vi "Chasis_Omni_Ultimate.vi"() -> ()   [LabVIEW 2010, in "Fiel Orientation Compass.lvrbt"]
uses:
  Fiel Orientation Compass.lvrbt
  <vilib>/NXT/HiTechnic/HiTechnic Controls/HiTechnic Port.ctl
  <vilib>/NXT/Block Support/NXT_InputPort.ctl
  <vilib>/NXT/NXTIO Xnodes/AddressXNode/NXTIOAddress.xnode
  <vilib>/NXT/Subs/MotorXNode.DC Motor Type.ctl
  Desktop/Teleop1.lvrbt_2012_01_27_1934/Teleop1/Teleop1.lvrbt
  <vilib>/NXT/Subs/MotorXNode.1DCMotor.ctl
  <vilib>/NXT/Subs/LVHSConnector.ctl
  <vilib>/NXT/NXTIO Xnodes/NXTIOXNode/NXTIO.xnode
  <vilib>/FTC/FTC Interpret Motor Power From Right X Axis.vi
  <vilib>/FTC/FTC Interpret Motor Power From Left Y Axis.vi
  <vilib>/FTC/FTC Interpret Motor Power From Left X Axis.vi
  <vilib>/NXT/Dual Mode Library/prims/inRangeAndCoerce/inRangeAndCoerce_float.vi
  <vilib>/NXT/NXTIO Xnodes/NXTIONodeSubVIs/TETRIX IO Move DC Motors.vi
panel:
  out "LEFT Y":i8
  out "LEFT X":i8
  out "y'":dbl
  out "x'":dbl
  out "INITIAL":dbl
  # "This VI was generated based on your configuration in the Remote Control Editor. You may modify the code as needed for your robot. To test this program for an FTC match, return to the Remote Control Editor, select the \"Run Program\" tab, and choose \"FTC Game\"."
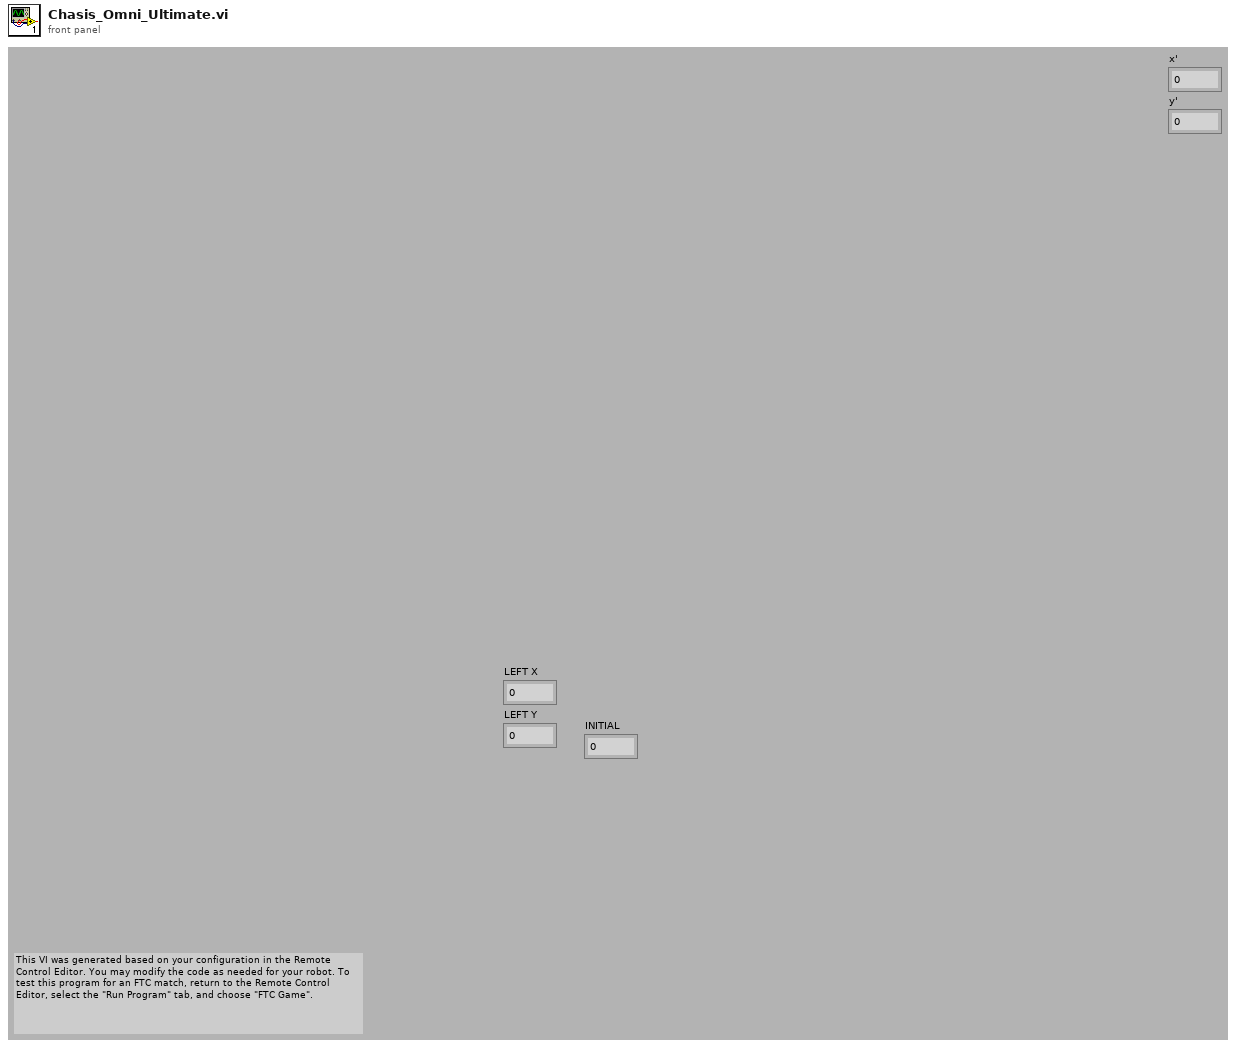
[diagram p1: front panel]
types:
  T1 = typedef "HiTechnic Port.ctl" = cluster{"Port":T2, "MUX Port":u8}
  T2 = typedef "NXT_InputPort.ctl" = u8
  T3 = typedef "LVHSConnector.ctl" = cluster{"Hardware":string, "Flattened String":string}
  T4 = typedef "FTC ControllerState.ctl" = cluster{"Left X":i8, "Left Y":i8, "Right X":i8, "Right Y":i8, "Button Encoding 9-12":u8, "Button Encoding 1-8":u8, "POV":T5}
  T5 = typedef "FTC POVState.ctl" = i8
  T6 = typedef "FTC ButtonEventType.ctl" = enum16{"Pressed", "Released"}
  T7 = cluster{"Button ID":enum16{"None", "Button 1", "Button 2", "Button 3", "Button 4", "Button 5", "Button 6", "Button 7", "Button 8", "Button 9", "Button 10", "Button 11", "Button 12", "POV Up", "POV Up Right", "POV Right", "POV Down Right", "POV Down", "POV Down Left", "POV Left", "POV Up Left"}, "Event Type":T6}[]
  T8 = enum16{"None", "Button 1", "Button 2", "Button 3", "Button 4", "Button 5", "Button 6", "Button 7", "Button 8", "Button 9", "Button 10", "Button 11", "Button 12", "POV Up", "POV Up Right", "POV Right", "POV Down Right", "POV Down", "POV Down Left", "POV Left", "POV Up Left"}
  T9 = typedef "MotorXNode.DC Motor Type.ctl" = enum16{"DC Motor"}
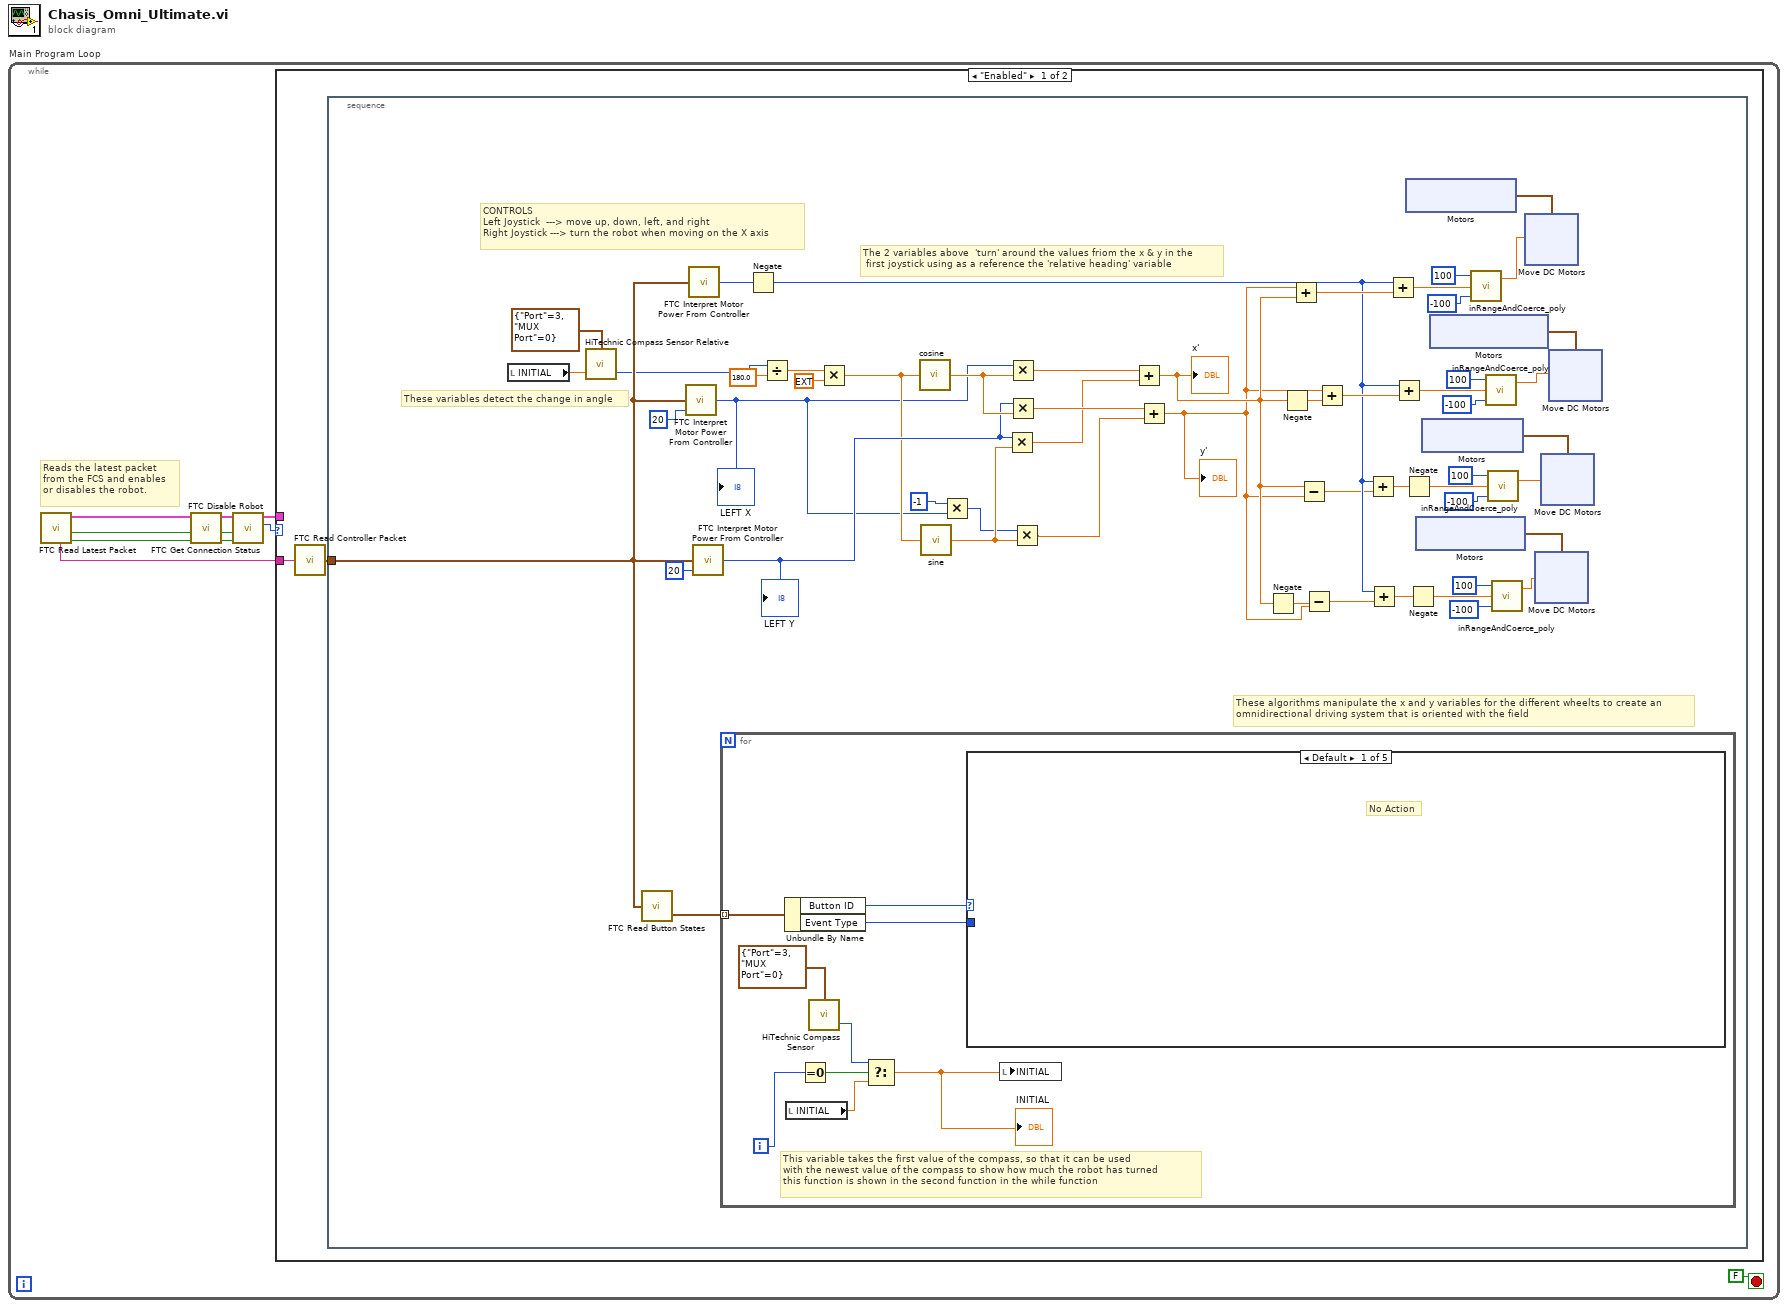
[diagram p0: block diagram]
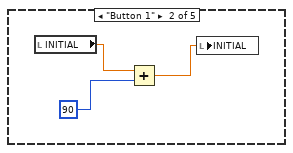
[diagram p2: hidden frame]
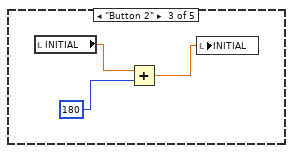
[diagram p3: hidden frame]
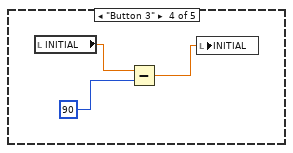
[diagram p4: hidden frame]
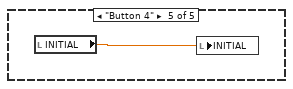
[diagram p5: hidden frame]
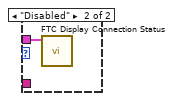
[diagram p6: hidden frame]
diagram:
  n1 = while "Main Program Loop" {
    stop <- FALSE stop-if-true
    # "Reads the latest packet\nfrom the FCS and enables\nor disables the robot."
    n2 = call <vilib>:"FTC Read Latest Packet.vi"() -> ("Packet Received?"=w8:bool, "Stopped?"=w5:bool, "NXT"=w7:T3, "Controller 1"=w9:string)  [unwired: 6 in, 2 out]
    n3 = call <vilib>:"FTC Get Connection Status.vi"("Packet Received?"=w8, "Stopped?"=w5, "NXT"=w7) -> ("Online?"=w2:bool, "Stopped?"=w3:bool, "NXT"=w4:T3)  [unwired: 5 in]
    n4 = call <vilib>:"FTC Disable Robot.vi"("Online?"=w2, "Stopped?"=w3, "NXT"=w4) -> ("Enabled?"=w6:enum16{"Disabled", "Enabled"}, "NXT"=w1:T3)  [unwired: 3 in]
    n5 = case "disableCase" shown="\"Enabled\"" w6 {
      tunnel: w9 -> [w12 _]
      tunnel: w1 -> [_ w121]
      frame "Enabled" {
        n6 = call <vilib>:"FTC Read Controller Packet.vi"("Packet"=w12) -> ("Controller State"=w11:T4)  [unwired: 4 in]
        n7 = stacked-sequence "controller1Actions" {
          tunnel: w11 -> [w65]
          frame #0 {
            # "These algorithms manipulate the x and y variables for the different wheelts to create an\nomnidirectional driving system that is oriented with the field"
            # "The 2 variables above  'turn' around the values friom the x & y in the\n\tfirst joystick using as a reference the 'relative heading' variable"
            # "These variables detect the change in angle"
            # "CONTROLS\nLeft Joystick  ---> move up, down, left, and right                   \nRight Joystick ---> turn the robot when moving on the X axis"
            n8 = local read "INITIAL"() -> (w43:dbl)
            n9 = call <vilib>:"HiTechnic Compass Sensor Relative.vi"("Target Heading (Degrees)"=w43, "Port/MUX"=T1 {"Port"=3, "MUX Port"=0}) -> ("Relative Heading (Degrees)"=w42:i32)  [unwired: 1 in, 1 out]
            n10 = call <vilib>:"FTC Read Button States.vi"("Controller State"=w65) -> ("Button Events"=w64:T7)  [unwired: 2 in, 1 out]
            n11 = call-poly <vilib>:"FTC Interpret Motor Power From Controller.vi"("Deadband (10)"=i8 20, "Controller State"=w65) -> ("Power"=w14:i8)  [unwired: 1 in]
            "LEFT X" <- w14
            n12 = call-poly <vilib>:"FTC Interpret Motor Power From Controller.vi"("Controller State"=w65) -> ("Power"=w63:i8)  [unwired: 2 in]
            n13 = call-poly <vilib>:"FTC Interpret Motor Power From Controller.vi"("Deadband (10)"=i8 20, "Controller State"=w65) -> ("Power"=w45:i8)  [unwired: 1 in]
            "LEFT Y" <- w45
            n14 = for "buttonAction" {
              tunnel: w64 -> [w108] mode=indexing
              i -> [w106]
              # "This variable takes the first value of the compass, so that it can be used\nwith the newest value of the compass to show how much the robot has turned \nthis function is shown in the second function in the while function"
              n15 = Unbundle By Name(w108) -> ("Button ID"=w110:T8, "Event Type"=w109:T6)
              n16 = local read "INITIAL"() -> (w105:dbl)
              n17 = Equal To 0?(x=w106) -> (x = 0?=w107:bool)
              n18 = call <vilib>:"HiTechnic Compass Sensor.vi"("Port/MUX"=T1 {"Port"=3, "MUX Port"=0}) -> ("Heading (degrees)"=w104:i16)  [unwired: 2 in, 1 out]
              n19 = Select(t=w104, s=w107, f=w105) -> (s? t:f=w102:dbl)
              "INITIAL" <- w102
              n20 = case "EventCase1" shown="Default" w110 {
                tunnel: w109 -> [_ _ _ _ _]
                frame Default {
                  # "No Action"
                }
                frame "Button 1" {
                  n21 = local read "INITIAL"() -> (w113:dbl)
                  n22 = Add(x=w113, y=90) -> (x+y=w112:dbl)
                  n23 = local write "INITIAL"(w112) -> ()
                }
                frame "Button 2" {
                  n24 = local read "INITIAL"() -> (w116:dbl)
                  n25 = Add(x=w116, y=180) -> (x+y=w115:dbl)
                  n26 = local write "INITIAL"(w115) -> ()
                }
                frame "Button 3" {
                  n27 = local read "INITIAL"() -> (w119:dbl)
                  n28 = Subtract(x=w119, y=90) -> (x-y=w118:dbl)
                  n29 = local write "INITIAL"(w118) -> ()
                }
                frame "Button 4" {
                  n30 = local read "INITIAL"() -> (w120:dbl)
                  n31 = local write "INITIAL"(w120) -> ()
                }
              }
              n32 = local write "INITIAL"(w102) -> ()
            }
            n33 = Negate(x=w63) -> (-x=w31:i8)
            n34 = Divide(x=w42, y=180.0) -> (x/y=w49:dbl)
            n35 = Multiply(x=w49, y=ext 3.1415926535897932385 ("Pi")) -> (x*y=w18:ext)
            n36 = call <vilib>:"cosine.vi"("x"=w18) -> ("cos(x)"=w47:sgl)
            n37 = call <vilib>:"sine.vi"("x"=w18) -> ("sin(x)"=w46:sgl)
            n38 = Multiply(x=-1, y=w14) -> (x*y=w13:i32)
            n39 = Multiply(x=w45, y=w46) -> (x*y=w17:sgl)
            n40 = Multiply(x=w14, y=w47) -> (x*y=w30:sgl)
            n41 = Multiply(x=w45, y=w47) -> (x*y=w29:sgl)
            n42 = Multiply(x=w13, y=w46) -> (x*y=w16:sgl)
            n43 = Add(x=w30, y=w17) -> (x+y=w26:sgl)
            "x'" <- w26
            n44 = Add(x=w29, y=w16) -> (x+y=w24:sgl)
            "y'" <- w24
            n45 = Negate(x=w26) -> (-x=w25:sgl)
            n46 = Negate(x=w26) -> (-x=w28:sgl)
            n47 = Add(x=w24, y=w26) -> (x+y=w33:sgl)
            n48 = Subtract(x=w26, y=w24) -> (x-y=w27:sgl)
            n49 = Subtract(x=w25, y=w24) -> (x-y=w23:sgl)
            n50 = Add(x=w24, y=w28) -> (x+y=w32:sgl)
            n51 = Add(x=w31, y=w27) -> (x+y=w21:sgl)
            n52 = Add(x=w31, y=w23) -> (x+y=w22:sgl)
            n53 = Add(x=w31, y=w33) -> (x+y=w54:sgl)
            n54 = Add(x=w31, y=w32) -> (x+y=w53:sgl)
            n55 = Negate(x=w21) -> (-x=w20:sgl)
            n56 = xnode "Motors"() -> ("DC Motor"=w41:cluster{"DC Motor":T9, "Address":i16})
            n57 = Negate(x=w22) -> (-x=w19:sgl)
            n58 = xnode "Motors"() -> ("DC Motor"=w35:cluster{"DC Motor":T9, "Address":i16})
            n59 = xnode "Motors"() -> ("DC Motor"=w37:cluster{"DC Motor":T9, "Address":i16})
            n60 = xnode "Motors"() -> ("DC Motor"=w39:cluster{"DC Motor":T9, "Address":i16})
            n61 = call-poly <vilib>:"inRangeAndCoerce_poly.vi"("lower limit"=-100, "x"=w54, "upper limit"=100) -> ("coerced(x)"=w40:dbl)  [unwired: 1 out]
            n62 = call-poly <vilib>:"inRangeAndCoerce_poly.vi"("lower limit"=-100, "x"=w53, "upper limit"=100) -> ("coerced(x)"=w38:dbl)  [unwired: 1 out]
            n63 = call-poly <vilib>:"inRangeAndCoerce_poly.vi"("lower limit"=-100, "x"=w20, "upper limit"=100) -> ("coerced(x)"=w36:dbl)  [unwired: 1 out]
            n64 = call-poly <vilib>:"inRangeAndCoerce_poly.vi"("lower limit"=-100, "x"=w19, "upper limit"=100) -> ("coerced(x)"=w34:dbl)  [unwired: 1 out]
            n65 = xnode "Move DC Motors"("Power/Speed 1"=w40, "Motors"=w41) -> ()  [unwired: 1 in, 1 out]
            n66 = xnode "Move DC Motors"("Power/Speed 1"=w34, "Motors"=w35) -> ()  [unwired: 1 in, 1 out]
            n67 = xnode "Move DC Motors"("Power/Speed 1"=w36, "Motors"=w37) -> ()  [unwired: 1 in, 1 out]
            n68 = xnode "Move DC Motors"("Power/Speed 1"=w38, "Motors"=w39) -> ()  [unwired: 1 in, 1 out]
          }
        }
      }
      frame "Disabled" {
        n69 = call <vilib>:"FTC Display Connection Status.vi"("NXT"=w121) -> ()  [unwired: 10 in, 1 out]
      }
    }
  }
